vi "ReadStream ServerStreamTemplate.vi"(8 "error in":errorcluster, 11 "Call ID in":T1) -> (0 "error out":errorcluster, 1 "Success":bool, 2 "Response Data":cluster{"Numeric":dbl}, 3 "Call ID":T1)   [LabVIEW 2020, in "MeasurementLink Pin Map Client.lvlib"]
uses:
  <vilib>/gRPC/LabVIEW gRPC Library/Shared/grpcId.ctl
  aea5dbbb-03a2-479b-ad95-94da4ee1cea9.vi
  c6b636f6-ccba-44e8-9d36-1b161804d74a.vi
  <vilib>/gRPC/LabVIEW gRPC Library/Shared/TranslateGrpcError.vi
  <vilib>/gRPC/LabVIEW gRPC Library/Shared/Wait On Occurence.vi
  <vilib>/gRPC/LabVIEW gRPC Library/Server API/Server/Get Server DLL Path.vi
  <vilib>/Utility/error.llb/Error Cluster From Error Code.vi
  <vilib>/Utility/error.llb/Simple Error Handler.vi
  MeasurementLink Pin Map Client.lvlib
  <vilib>/gRPC/LabVIEW gRPC Library/grpc-lvsupport-release.lvlib
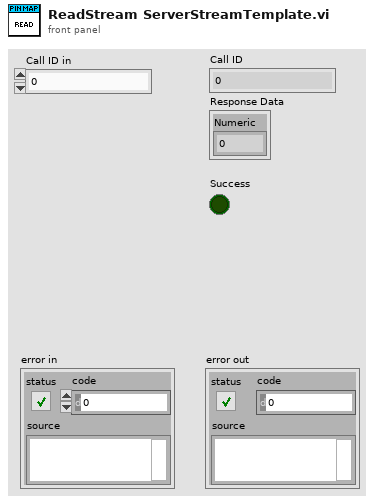
[diagram p1: front panel]
types:
  T1 = typedef "grpc-lvsupport-release.lvlib/grpcId.ctl" = u64
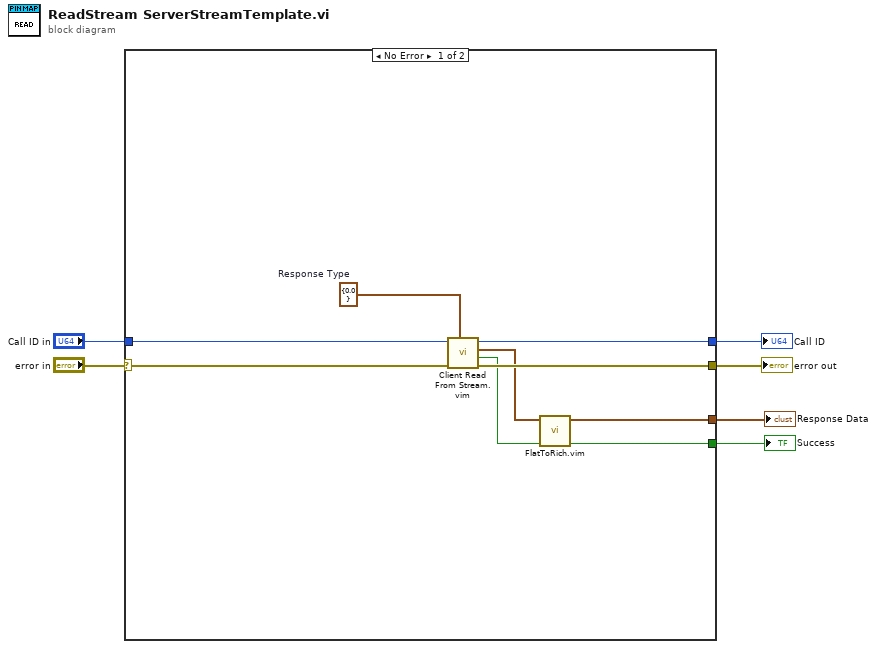
[diagram p0: block diagram]
diagram:
  n1 = case shown="No Error" "error in" {
    selector: "error in" -> [w14 w15]
    tunnel: [w13 w15] -> w5
    tunnel: "Call ID in" -> [w12 w16]
    tunnel: [w10 w16] -> w3
    tunnel: [w7 _] -> w2
    tunnel: [w11 _] -> w1
    frame No Error {
      w9 = cluster{"Numeric":dbl} {"Numeric"=0.0}  # Response Type
      n2 = call "Client Read From Stream.vim"("Response Type"=w9, "error in"=w14, "Call ID in"=w12) -> ("error out"=w13:errorcluster, "Success"=w11:bool, "Response Data"=w8:cluster{"Numeric":dbl}, "Call ID out"=w10:u64)  [unwired: 5 in]
      n3 = call "FlatToRich.vim"("InputCluster"=w8) -> ("OutputCluster"=w7:cluster{"Numeric":dbl})  [unwired: 10 in]
    }
    frame Error {
    }
  }
  "error out" <- w5
  "Call ID" <- w3
  "Response Data" <- w2
  "Success" <- w1
